vi "Periodic Tasks.vi"(8 "error in":errorcluster) -> ()   [LabVIEW 2013]
doc: "This VI runs in parallel to other tasks. It can contain as many user-defined periodic loops as you need. These can carry out PID or other sorts of timed response."
uses:
  <vilib>/Rock Robotics/SystemInterfaces/DIO/FPGA_DIOChannel.ctl
  <vilib>/Rock Robotics/SystemInterfaces/DIO/FPGA_DIORelayChannel.ctl
  <vilib>/Rock Robotics/SystemInterfaces/Utilities/FPGA_UtilitiesLED Source.ctl
  <vilib>/Rock Robotics/SystemInterfaces/Utilities/FPGA_UtilitiesLED State.ctl
  Robot Global Data.vi
panel:
  out "error out":errorcluster
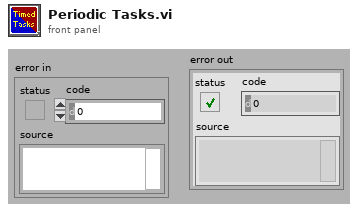
[diagram p1: front panel]
types:
  T1 = typedef "FPGA_DIORelayChannel.ctl" = enum8{"Relay 1", "Relay 2", "Relay 3", "Relay 4", "Relay 5", "Relay 6", "Relay 7", "Relay 8", "Invalid"}
  T2 = typedef "FPGA_DIOChannel.ctl" = enum8{"DIO 1", "DIO 2", "DIO 3", "DIO 4", "DIO 5", "DIO 6", "DIO 7", "DIO 8", "DIO 9", "DIO 10", "DIO 11", "DIO 12", "DIO 13", "DIO 14", "Invalid"}
  T3 = typedef "WPI_DigitalInputDevRef.ctl" = cluster{"DevStatus":errorcluster, "DIO Channel":T2, "Digital Module":T4}
  T4 = typedef "FPGA_TypedefDigitalModule.ctl" = enum16{"Digital Module 1", "Digital Module 2"}
  T5 = typedef "FPGA_UtilitiesLED State.ctl" = enum16{"Off", "On", "Toggle"}
  T6 = typedef "FPGA_UtilitiesLED Source.ctl" = enum16{"User LED", "FPGA LED"}
  T7 = typedef "WPI_CompressorDevRef.ctl" = cluster{"DevStatus":errorcluster, "DigitalInputDevRef":T3, "RelayDevRef":T8}
  T8 = typedef "WPI_RelayDevRef.ctl" = cluster{"DevStatus":errorcluster, "Relay Channel":T1, "Digital Module":T4, "Relay Direction":T9}
  T9 = typedef "WPI_RelayDirection.ctl" = enum16{"Both directions", "Forward only", "Reverse only"}
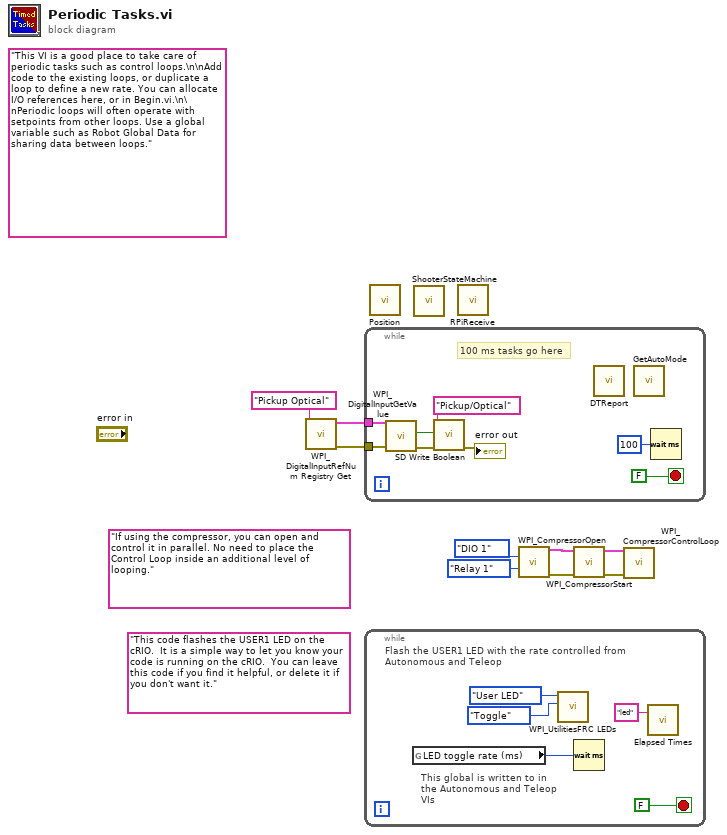
[diagram p0: block diagram]
diagram:
  (unwired) "If using the compressor, you can open and control it in parallel. No need to place the Control Loop inside an additional level of looping."
  (unwired) "This code flashes the USER1 LED on the cRIO.  It is a simple way to let you know your code is running on the cRIO.  You can leave this code if you find it helpful, or delete it if you don't want it."
  (unwired) "This VI is a good place to take care of periodic tasks such as control loops.\n\nAdd code to the existing loops, or duplicate a loop to define a new rate. You can allocate I/O references here, or in Begin.vi.\n\nPeriodic loops will often operate with setpoints from other loops. Use a global variable such as Robot Global Data for sharing data between loops."
  n1 = call <vilib>:"WPI_DigitalInputRefNum Registry Get.vi"("refnum name"="Pickup Optical") -> ("error out"=w1:errorcluster, "DigitalInputDevRef"=w2:T3)  [unwired: 9 in]
  n2 = while {
    tunnel: w2 -> [w15]
    tunnel: w1 -> [w14]
    stop <- FALSE stop-if-true
    # "100 ms tasks go here"
    n3 = call <vilib>:"WPI_DigitalInputGetValue.vi"("error in (no error)"=w14, "DigitalInputDevRef"=w15) -> ("error out"=w13:errorcluster, "Value"=w11:bool)  [unwired: 7 in, 1 out]
    n4 = call <vilib>:"SD Write Boolean.vi"("error in"=w13, "Boolean"=w11, "Name"="Pickup/Optical") -> ("error out"=→"error out":errorcluster)  [unwired: 7 in, 1 out]
    n5 = call "DTReport.vi"() -> ()  [unwired: 12 in]
    n6 = call "GetAutoMode.vi"() -> ()  [unwired: 12 in]
    n7 = Wait (ms)(milliseconds to wait=u32 100) -> ()  [unwired: 1 out]
  }
  n8 = while {
    stop <- FALSE stop-if-true
    # "This global is written to in the Autonomous and Teleop VIs"
    # "Flash the USER1 LED with the rate controlled from Autonomous and Teleop"
    n9 = global read "Robot Global Data.vi" "LED toggle rate (ms)"() -> (w19:u32)
    n10 = call <vilib>:"WPI_UtilitiesFRC LEDs.vi"("State"=FPGA_UtilitiesLED_State."Toggle", "LED Type"=FPGA_UtilitiesLED_Source."User LED") -> ()  [unwired: 1 in, 9 out]
    n11 = Wait (ms)(milliseconds to wait=w19) -> ()  [unwired: 1 out]
    n12 = call "Elapsed Times.vi"("Call Name"="led") -> ()  [unwired: 2 in, 1 out]
  }
  n13 = call "Position.vi"() -> ()  [unwired: 12 in]
  n14 = call "ShooterStateMachine.vi"() -> ()  [unwired: 12 in]
  n15 = call "RPiReceive.vi"() -> ()  [unwired: 12 in]
  n16 = call <vilib>:"WPI_CompressorOpen.vi"("Pressure Switch DIO Channel"=FPGA_DIOChannel."DIO 1", "Relay Channel"=FPGA_DIORelayChannel."Relay 1") -> ("CompressorDevRef"=w7:T7, "error out"=w6:errorcluster)  [unwired: 12 in]
  n17 = call <vilib>:"WPI_CompressorStart.vi"("error in (no error)"=w6, "CompressorDevRef"=w7) -> ("error out"=w9:errorcluster, "CompressorDevRef"=w8:T7)  [unwired: 8 in]
  n18 = call <vilib>:"WPI_CompressorControlLoop.vi"("error in (no error)"=w9, "CompressorDevRef"=w8) -> ()  [unwired: 10 in]
